vi "Send Stop Message.vi"(7 "Emergency Stop? (F)":bool, 8 "error in (no error)":errorcluster, 11 "API-Reference in":refnum<data-value>) -> (0 "error out":errorcluster, 3 "API-Reference out":refnum<data-value>)   [LabVIEW 2018, in "Actor.lvclass"]
uses:
  Actor.lvclass
  API-Data.ctl
  Stopped.ctl
  Message-Enqueue Refs.ctl
  Stop.ctl
  Launch.ctl
  Did Initialize.ctl
  <vilib>/event_ctls.llb/usereventprio.ctl
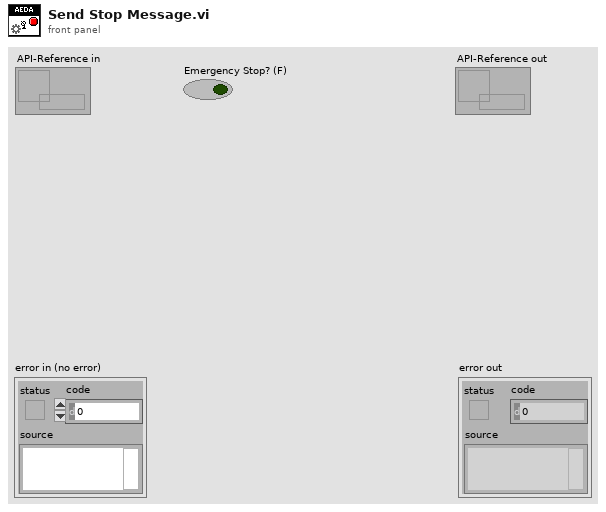
[diagram p1: front panel]
types:
  T1 = typedef "Actor.lvclass/Stop.ctl" = enum16{"Normal", "Emergency"}
  T2 = typedef "usereventprio.ctl" = enum32{"high priority", "normal priority"}
  T3 = typedef "Actor.lvclass/API-Data.ctl" = cluster{"Launch":refnum<notifier>, "Did Stop Enqueuer":refnum<user-event>, "Message Enqueuers":T4, "Stopped Reg":refnum<event-registration>}
  T4 = typedef "Actor.lvclass/Message-Enqueue Refs.ctl" = cluster{"Stop":refnum<user-event>, "Launch":refnum<user-event>, "Did Initialize":refnum<user-event>}
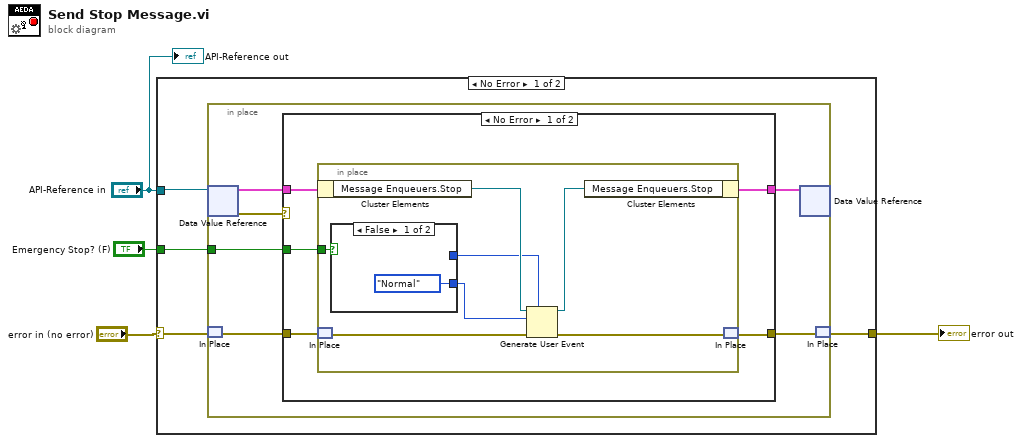
[diagram p0: block diagram]
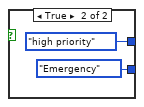
[diagram p2: hidden frame]
diagram:
  n1 = case shown="No Error" "error in (no error)" {
    selector: "error in (no error)" -> [w8 w32]
    tunnel: [w7 w32] -> w2
    tunnel: "API-Reference in" -> [w5 _]
    tunnel: "Emergency Stop? (F)" -> [w6 _]
    frame No Error {
      n2 = in-place {
        in-place-border: w6 -> [w9]
        n3 = in-place-dvr #1(w5) -> (w13:T3, w14:errorcluster)
        n4 = in-place-match #2(w8) -> (w11:errorcluster)
        n5 = case shown="No Error" w14 {
          selector: w14 -> [_ w31]
          tunnel: w13 -> [w17 w30]
          tunnel: [w15 w30] -> w12
          tunnel: w11 -> [w19 _]
          tunnel: [w18 w31] -> w10
          tunnel: w9 -> [w16 _]
          frame No Error {
            n6 = in-place {
              in-place-border: w16 -> [w24]
              n7 = in-place-cluster #3(w17) -> ("Message Enqueuers.Stop"=w25:refnum<user-event>)
              n8 = in-place-match #4(w19) -> (w26:errorcluster)
              n9 = case shown="False" w24 {
                tunnel: [Stop."Normal" ("Stop") Stop."Emergency" ("Stop")] -> w22
                tunnel: [_ usereventprio."high priority" ("priority (normal)")] -> w21
                frame False {
                }
                frame True {
                }
              }
              n10 = Generate User Event(priority (normal)=w21, user event=w25, event data cluster=w22, error in=w26) -> (user event out=w23:refnum<user-event>, error out=w20:errorcluster)
              n11 = in-place-cluster #3("Message Enqueuers.Stop"=w23) -> (w15:T3)
              n12 = in-place-match #4(w20) -> (w18:errorcluster)
            }
          }
          frame Error {
          }
        }
        n13 = in-place-dvr #1(w12) -> ()  [unwired: 2 out]
        n14 = in-place-match #2(w10) -> (w7:errorcluster)
      }
    }
    frame Error {
    }
  }
  "error out" <- w2
  "API-Reference out" <- "API-Reference in"
